vi "CoerseNumericType.vi"(7 "Numeric Variant in":variant, 8 "error in (no error)":errorcluster, 11 "Numeric":cxt) -> (0 "error out":errorcluster, 3 "Numeric Variant out":variant)   [LabVIEW 2020]
uses:
  <vilib>/Utility/Data Type/NI_Data Type.lvlib
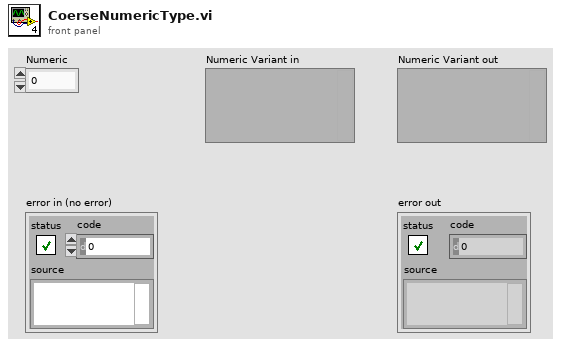
[diagram p1: front panel]
types:
  T1 = typedef "LVNumericRepresentation.ctl" = enum32{"Extended Precision", "Double Precision", "Single Precision", "Long", "Word", "Byte", "Unsigned Long", "Unsigned Word", "Unsigned Byte", "Complex Extended", "Complex Double", "Complex Single", "Quad", "Unsigned Quad", "Fixed-Point"}
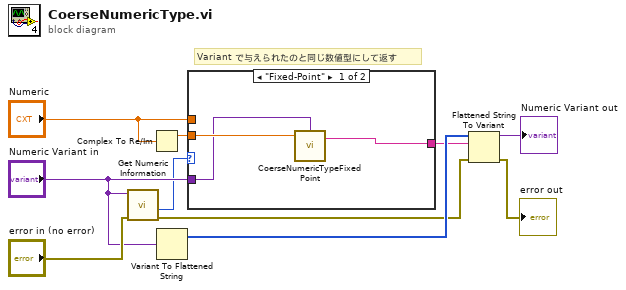
[diagram p0: block diagram]
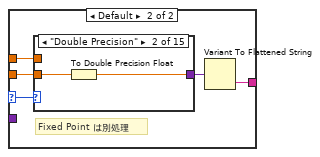
[diagram p2: hidden frame]
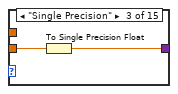
[diagram p4: hidden frame]
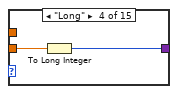
[diagram p5: hidden frame]
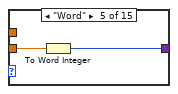
[diagram p6: hidden frame]
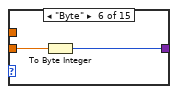
[diagram p7: hidden frame]
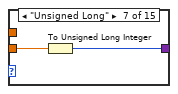
[diagram p8: hidden frame]
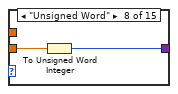
[diagram p9: hidden frame]
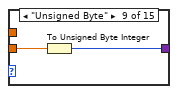
[diagram p10: hidden frame]
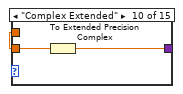
[diagram p11: hidden frame]
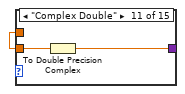
[diagram p12: hidden frame]
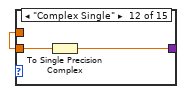
[diagram p13: hidden frame]
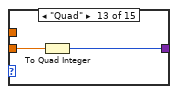
[diagram p14: hidden frame]
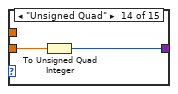
[diagram p15: hidden frame]
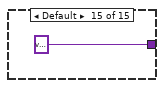
[diagram p16: hidden frame]
diagram:
  # "Variant で与えられたのと同じ数値型にして返す"
  n1 = call <vilib>:"Get Numeric Information.vi"("error in (no error)"="error in (no error)", "variant"="Numeric Variant in") -> ("error out"=w7:errorcluster, "representation"=w1:T1)  [unwired: 6 in, 2 out]
  n2 = Complex To Re/Im(x + iy="Numeric") -> (x=w4:ext)  [unwired: 1 out]
  n3 = Variant To Flattened String(Variant="Numeric Variant in") -> (1:w9:i16[])  [unwired: 1 out]
  n4 = case shown="\"Fixed-Point\"" w1 {
    selector: w1 -> [_ w14]
    tunnel: [w13 w17] -> w5
    tunnel: w4 -> [w12 w16]
    tunnel: "Numeric" -> [_ w15]
    tunnel: "Numeric Variant in" -> [w11 _]
    frame "Fixed-Point" {
      n5 = call "CoerseNumericTypeFixedPoint.vi"("Numeric Variant in"=w11, "Numeric"=w12) -> ("Encoded"=w13:string)  [unwired: 3 in]
    }
    frame Default {
      # "Fixed Point は別処理"
      n6 = case shown="\"Double Precision\"" w14 {
        tunnel: w16 -> [w19 w21 w23 w25 w27 w29 w31 w33 w35 _ _ _ w43 w45 _]
        tunnel: [w19 w20 w22 w24 w26 w28 w30 w32 w34 w37 w39 w41 w42 w44 variant ("Numeric Variant out")] -> w18
        tunnel: w15 -> [_ _ _ _ _ _ _ _ _ w36 w38 w40 _ _ _]
        frame "Extended Precision" {
        }
        frame "Double Precision" {
          n7 = To Double Precision Float(number=w21) -> (double precision float=w20:dbl)
        }
        frame "Single Precision" {
          n8 = To Single Precision Float(number=w23) -> (single precision float=w22:sgl)
        }
        frame "Long" {
          n9 = To Long Integer(number=w25) -> (32bit integer=w24:i32)
        }
        frame "Word" {
          n10 = To Word Integer(number=w27) -> (16bit integer=w26:i16)
        }
        frame "Byte" {
          n11 = To Byte Integer(number=w29) -> (8bit integer=w28:i8)
        }
        frame "Unsigned Long" {
          n12 = To Unsigned Long Integer(number=w31) -> (unsigned 32bit integer=w30:u32)
        }
        frame "Unsigned Word" {
          n13 = To Unsigned Word Integer(number=w33) -> (unsigned 16bit integer=w32:u16)
        }
        frame "Unsigned Byte" {
          n14 = To Unsigned Byte Integer(number=w35) -> (unsigned 8bit integer=w34:u8)
        }
        frame "Complex Extended" {
          n15 = To Extended Precision Complex(1:w36) -> (0:w37:cxt)
        }
        frame "Complex Double" {
          n16 = To Double Precision Complex(1:w38) -> (0:w39:cdb)
        }
        frame "Complex Single" {
          n17 = To Single Precision Complex(1:w40) -> (0:w41:csg)
        }
        frame "Quad" {
          n18 = To Quad Integer(1:w43) -> (0:w42:i64)
        }
        frame "Unsigned Quad" {
          n19 = To Unsigned Quad Integer(1:w45) -> (0:w44:u64)
        }
        frame Default {
        }
      }
      n20 = Variant To Flattened String(Variant=w18) -> (data string=w17:string)  [unwired: 1 out]
    }
  }
  n21 = Flattened String To Variant(4:w7, 6:w5, 7:w9) -> (0:→"error out":errorcluster, 3:→"Numeric Variant out":variant)
